vi "软触发子程序.vi"(4 "触发":bool, 5 "预触发长度":i32, 6 "task/channels in":refnum<k21>, 7 "阈值":dbl format="%#_13g", 8 "error in (no error)":errorcluster, 9 "Dummy Output Data":waveform(dbl)[](graph), 10 "激振信号":waveform(dbl)[](graph), 11 "激振通道":i32) -> (0 "error out":errorcluster, 1 "task out":refnum<k21>, 2 "ÏìÓ¦ÐÅº3":waveform(dbl)[](graph), 3 "模拟触发":bool)   [LabVIEW 2014]
uses:
  <vilib>/DAQmx/read.llb/DAQmx Read (Analog 1D Wfm NChan NSamp).vi
  <vilib>/Waveform/WDTOps.llb/WDT Number of Waveform Samples DBL.vi
  <vilib>/DAQmx/miscellaneous.llb/DAQmx Fill In Error Info.vi
  <vilib>/Waveform/WDTOps.llb/WDT Get Waveform Subset DBL.vi
  <vilib>/Waveform/WDTOps.llb/WDT Append Waveforms DBL.vi
panel:
  out "激振信号 2":dbl[](graph)
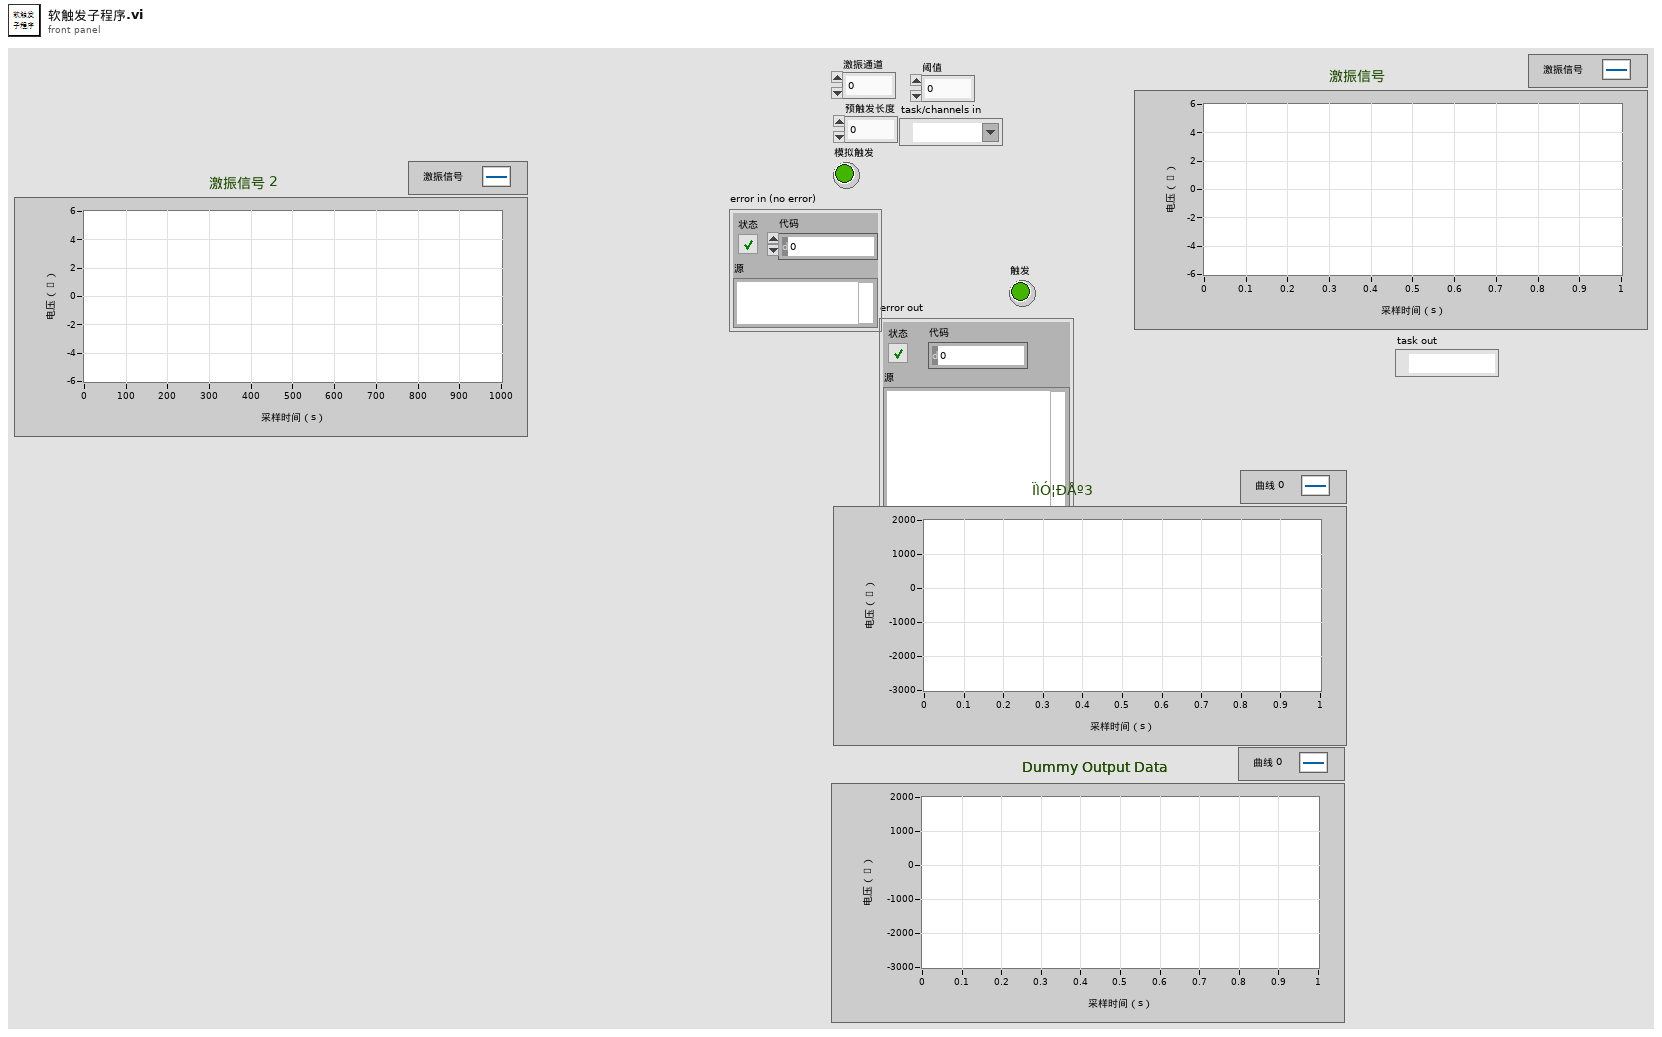
[diagram p1: front panel]
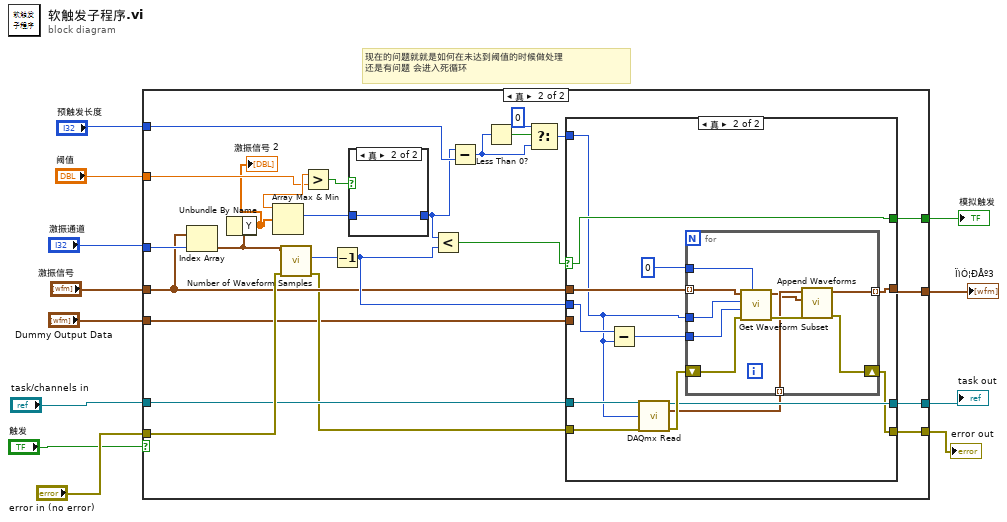
[diagram p0: block diagram]
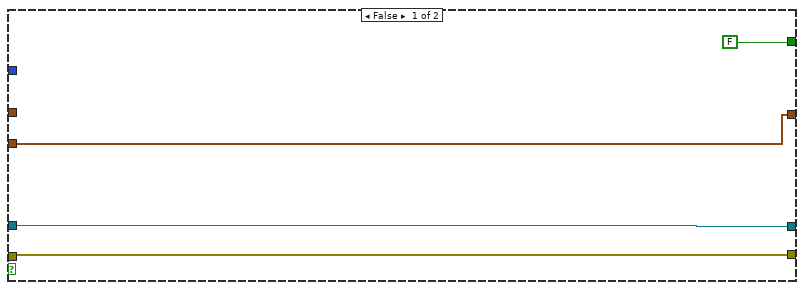
[diagram p2: hidden frame]
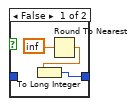
[diagram p3: hidden frame]
diagram:
  # "现在的问题就就是如何在未达到阈值的时候做处理\n还是有问题 会进入死循环"
  n1 = case shown="真" "触发" {
    tunnel: "激振信号" -> [_ w29]
    tunnel: "激振通道" -> [_ w41]
    tunnel: "error in (no error)" -> [w15 w38]
    tunnel: "阈值" -> [_ w36]
    tunnel: "预触发长度" -> [_ w35]
    tunnel: "task/channels in" -> [w16 w27]
    tunnel: [w16 w25] -> w5
    tunnel: [w15 w24] -> w6
    tunnel: [w14 w23] -> w4
    tunnel: "Dummy Output Data" -> [w14 w21]
    tunnel: [FALSE w22] -> w1
    frame False {
    }
    frame True {
      n2 = Index Array(array=w29, index=w41) -> (element=w40:waveform(dbl))
      n3 = Unbundle By Name(w40) -> ("Y"=w17:dbl[])
      "激振信号 2" <- w17
      n4 = Array Max & Min(array=w17) -> (max value=w37:dbl, max index (indices)=w19:i32)  [unwired: 2 out]
      n5 = call-poly <vilib>:"Number of Waveform Samples.vi"("error in (no error)"=w38, "waveform in"=w40) -> ("error out"=w26:errorcluster, "number of samples"=w39:i32)  [unwired: 7 in, 1 out]
      n6 = Greater?(x=w37, y=w36) -> (0:w20:bool)
      n7 = Decrement(x=w39) -> (x-1=w30:i32)
      n8 = case shown="真" w20 {
        tunnel: w19 -> [_ w45]
        tunnel: [w42 w45] -> w18
        frame False {
          n9 = Round To Nearest(number=inf) -> (nearest integer value=w43:dbl)
          n10 = To Long Integer(number=w43) -> (32bit integer=w42:i32)
        }
        frame True {
        }
      }
      n11 = Less?(x=w18, y=w30) -> (x < y?=w31:bool)
      n12 = Subtract(x=w18, y=w35) -> (x-y=w33:i32)
      n13 = Less Than 0?(x=w33) -> (x < 0?=w34:bool)
      n14 = Select(t=0, s=w34, f=w33) -> (s? t:f=w28:i32)
      n15 = case shown="真" w31 {
        selector: w31 -> [w47 w53]
        tunnel: w30 -> [_ w62]
        tunnel: w29 -> [_ w57]
        tunnel: w28 -> [_ w50]
        tunnel: w27 -> [w49 w61]
        tunnel: w26 -> [w48 w60]
        tunnel: [w49 w56] -> w25
        tunnel: [w48 w55] -> w24
        tunnel: [w46 w54] -> w23
        tunnel: [w47 w53] -> w22
        tunnel: w21 -> [w46 _]
        frame False {
        }
        frame True {
          n16 = Subtract(x=w62, y=w50) -> (x-y=w58:i32)
          n17 = call-poly <vilib>:"DAQmx Read.vi"("task/channels in"=w61, "number of samples per channel"=w50, "error in"=w60) -> ("task out"=w56:refnum<k21>, "data"=w52:waveform(dbl)[], "error out"=w59:errorcluster)  [unwired: 10 in]
          n18 = for {
            shift-right: [w66] -> w55
            shift-left: w59 -> [w68]
            tunnel: w58 -> [w70]
            tunnel: w50 -> [w71]
            tunnel: w57 -> [w72] mode=indexing
            tunnel: [w69] -> w54 mode=indexing
            tunnel: w52 -> [w64] mode=indexing
            tunnel: 0 -> [w65]
            n19 = call-poly <vilib>:"Get Waveform Subset.vi"("start/duration format"=w65, "error in (no error)"=w68, "duration"=w70, "start samples/time"=w71, "waveform in"=w72) -> ("error out"=w67:errorcluster, "waveform out"=w63:waveform(dbl))  [unwired: 1 in, 2 out]
            n20 = call-poly <vilib>:"Append Waveforms.vi"("error in (no error)"=w67, "waveform B"=w63, "waveform A"=w64) -> ("error out"=w66:errorcluster, "waveform out"=w69:waveform(dbl))  [unwired: 7 in]
          }
        }
      }
    }
  }
  "error out" <- w6
  "task out" <- w5
  "ÏìÓ¦ÐÅº3" <- w4
  "模拟触发" <- w1
